vi "Calc total coins.vi"(10 "Coins":bool[](array[boolean]), 11 "All my coins":dbl[](array[numeric])) -> (3 "Total (£)":dbl)   [LabVIEW 2018]
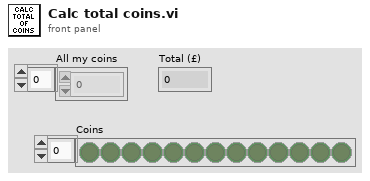
[diagram p1: front panel]
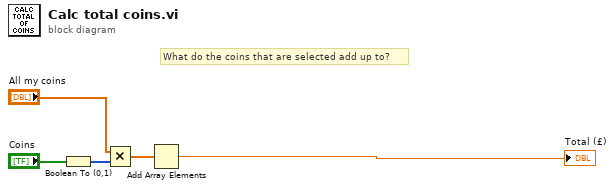
[diagram p0: block diagram]
diagram:
  # "What do the coins that are selected add up to?"
  n1 = Boolean To (0,1)(Boolean="Coins") -> (0, 1=w4:i16[])
  n2 = Multiply(x="All my coins", y=w4) -> (x*y=w3:dbl[])
  n3 = Add Array Elements(numeric array=w3) -> (sum=→"Total (£)":dbl)
